vi "test_libssh2_channel_receive_window_adjust2.vi"() -> ()   [LabVIEW 2013, in "libssh2_integration_tests.lvlib"]
uses:
  libssh2_integration_tests.lvlib
  <vilib>/addons/_JKI Toolkits/Caraya/classes/Test/Test.lvclass
  support/support.lvlib
  libssh2/libssh2.lvlib
  <vilib>/addons/_JKI Toolkits/Caraya/classes/Assert/Assert.lvclass
panel:
  out "error out":errorcluster
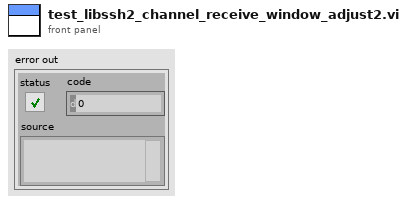
[diagram p1: front panel]
types:
  T1 = typedef "libssh2.lvlib/Session Refnum.ctl" = refnum<k1>
  T2 = typedef "libssh2.lvlib/Channel Refnum.ctl" = refnum<k1>
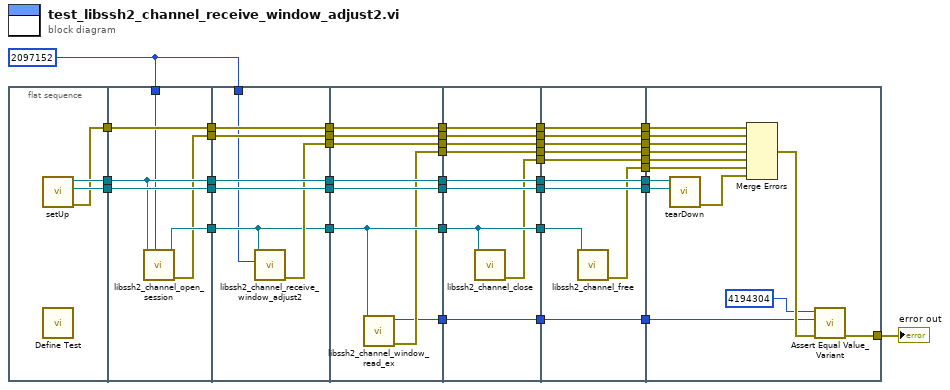
[diagram p0: block diagram]
diagram:
  w1 = u32 2097152 ("window_size (2 MiB)")
  n1 = flat-sequence {
    tunnel: [w45] -> w42
    tunnel: [w44] -> w41
    tunnel: [w43] -> w40
    tunnel: w42 -> [w50]
    tunnel: w41 -> [w51]
    tunnel: [w50] -> w39
    tunnel: [w51] -> w38
    tunnel: [w49] -> w37
    tunnel: w40 -> [w48]
    tunnel: [w48] -> w36
    tunnel: [w47] -> w35
    tunnel: w1 -> [w46]
    tunnel: w39 -> [w58]
    tunnel: [w58] -> w34
    tunnel: w38 -> [w57]
    tunnel: [w57] -> w33
    tunnel: w37 -> [w53]
    tunnel: [w53] -> w32
    tunnel: w36 -> [w56]
    tunnel: [w56] -> w31
    tunnel: w35 -> [w55]
    tunnel: [w55] -> w30
    tunnel: [w54] -> w29
    tunnel: w1 -> [w52]
    tunnel: w34 -> [w66]
    tunnel: [w66] -> w28
    tunnel: w33 -> [w65]
    tunnel: [w65] -> w27
    tunnel: w32 -> [w61]
    tunnel: [w61] -> w26
    tunnel: w31 -> [w64]
    tunnel: [w64] -> w25
    tunnel: w30 -> [w63]
    tunnel: [w63] -> w24
    tunnel: w29 -> [w62]
    tunnel: [w62] -> w23
    tunnel: [w60] -> w22
    tunnel: [w59] -> w21
    tunnel: w28 -> [w75]
    tunnel: w27 -> [w74]
    tunnel: w26 -> [w73]
    tunnel: [w75] -> w20
    tunnel: [w74] -> w19
    tunnel: [w67] -> w18
    tunnel: [w73] -> w17
    tunnel: [w72] -> w16
    tunnel: w25 -> [w71]
    tunnel: [w71] -> w15
    tunnel: w24 -> [w70]
    tunnel: [w70] -> w14
    tunnel: w23 -> [w69]
    tunnel: [w69] -> w13
    tunnel: w22 -> [w68]
    tunnel: [w68] -> w12
    tunnel: w21 -> [w67]
    tunnel: w20 -> [w85]
    tunnel: w19 -> [w84]
    tunnel: w18 -> [w83]
    tunnel: w17 -> [w82]
    tunnel: [w85] -> w11
    tunnel: [w84] -> w10
    tunnel: [w83] -> w9
    tunnel: [w81] -> w8
    tunnel: w16 -> [w80]
    tunnel: [w80] -> w7
    tunnel: w15 -> [w79]
    tunnel: [w79] -> w6
    tunnel: w14 -> [w78]
    tunnel: [w78] -> w5
    tunnel: w13 -> [w77]
    tunnel: [w77] -> w4
    tunnel: w12 -> [w76]
    tunnel: [w76] -> w3
    tunnel: w11 -> [w98]
    tunnel: w10 -> [w97]
    tunnel: w9 -> [w87]
    tunnel: [w96] -> w2
    tunnel: w8 -> [w94]
    tunnel: w7 -> [w93]
    tunnel: w6 -> [w92]
    tunnel: w5 -> [w90]
    tunnel: w4 -> [w89]
    tunnel: w3 -> [w88]
    frame #0 {
      n2 = call "setUp.vi"() -> ("error out"=w43:errorcluster, "connection ID"=w44:refnum<k5>, "session"=w45:T1)  [unwired: 9 in]
      n3 = call <vilib>:"Define Test.vi"() -> ()  [unwired: 10 in, 2 out]
    }
    frame #1 {
      n4 = call "libssh2_channel_open_session.vi"("window_size (2 MiB)"=w46, "session"=w50) -> ("error out"=w47:errorcluster, "channel"=w49:T2)  [unwired: 8 in]
    }
    frame #2 {
      n5 = call "libssh2_channel_receive_window_adjust2.vi"("adjustment"=w52, "channel"=w53) -> ("error out"=w54:errorcluster)  [unwired: 8 in, 1 out]
    }
    frame #3 {
      n6 = call "libssh2_channel_window_read_ex.vi"("channel"=w61) -> ("error out"=w60:errorcluster, "remaining read window"=w59:u32)  [unwired: 7 in, 2 out]
    }
    frame #4 {
      n7 = call "libssh2_channel_close.vi"("channel"=w73) -> ("error out"=w72:errorcluster)  [unwired: 10 in]
    }
    frame #5 {
      n8 = call "libssh2_channel_free.vi"("channel"=w82) -> ("error out"=w81:errorcluster)  [unwired: 10 in]
    }
    frame #6 {
      n9 = call "tearDown.vi"("connection ID"=w97, "session"=w98) -> ("error out"=w95:errorcluster)  [unwired: 9 in]
      n10 = Merge Errors(w92, w90, w89, w88, w93, w94, w95) -> (w91:errorcluster)
      n11 = call <vilib>:"Assert Equal Value_Variant.vi"("error in (no error)"=w91, "Y"=w87, "X"=u32 4194304 ("adjustment")) -> ("error out"=w96:errorcluster)  [unwired: 7 in, 1 out]
    }
  }
  "error out" <- w2
